vi "MDO32_2-2-Channel_V2.vi"() -> ()   [LabVIEW 2015]
uses:
  <vilib>/Utility/file.llb/Write Delimited Spreadsheet (string).vi
  <vilib>/Utility/file.llb/Write Delimited Spreadsheet (DBL).vi
panel:
  out "Iteration Running":bool
  out "Sample 4 Saved":bool
  out "Sample 3 Saved":bool
  out "Sample 2 Saved":bool
  out "Sample 1 Saved":bool
  in  "Test Name":string="TEST_NAME"
  in  "File Path Control":path
  in  "Temperature cDAQ1Mod1":tag="cDAQ1Mod1"
  in  "Oscilliscope MDO32_2":refnum<visa-resource-name>="MDO32_2"
  out "Iteration Number":i32
  out "Start Time and Date":timestamp
  in  "Stop":bool
  in  "Wait Time (s)":dbl=10.0
  in  "Oscilliscope MDO32_1":refnum<visa-resource-name>="MDO32_1"
  # "Test Settings"
  # "Test Info and Status"
  # "ENSURE THAT USBs ARE PLUGGED IN. DATA WILL NOT SAVE WITHOUT IT.\n\nUSB 1 GOES INTO OSC 1\nUSB 2 GOES INTO OSC 2\n\nPROGRAM WILL GET STUCK IF DEVICES ARE NOT CONNECTED OR SET UP APPROPRIATELY"
  # "CLICK STOP BUTTON ONLY ONCE\nIt takes time to stop as the loop needs to complete the current iteration and one more full iteration before it stops."
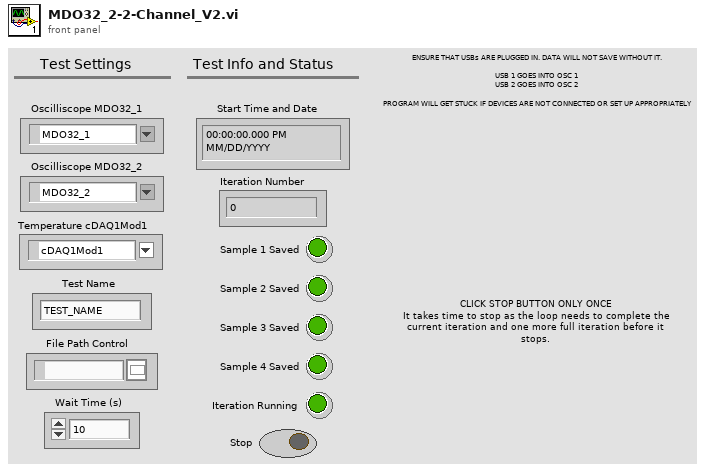
[diagram p1: front panel]
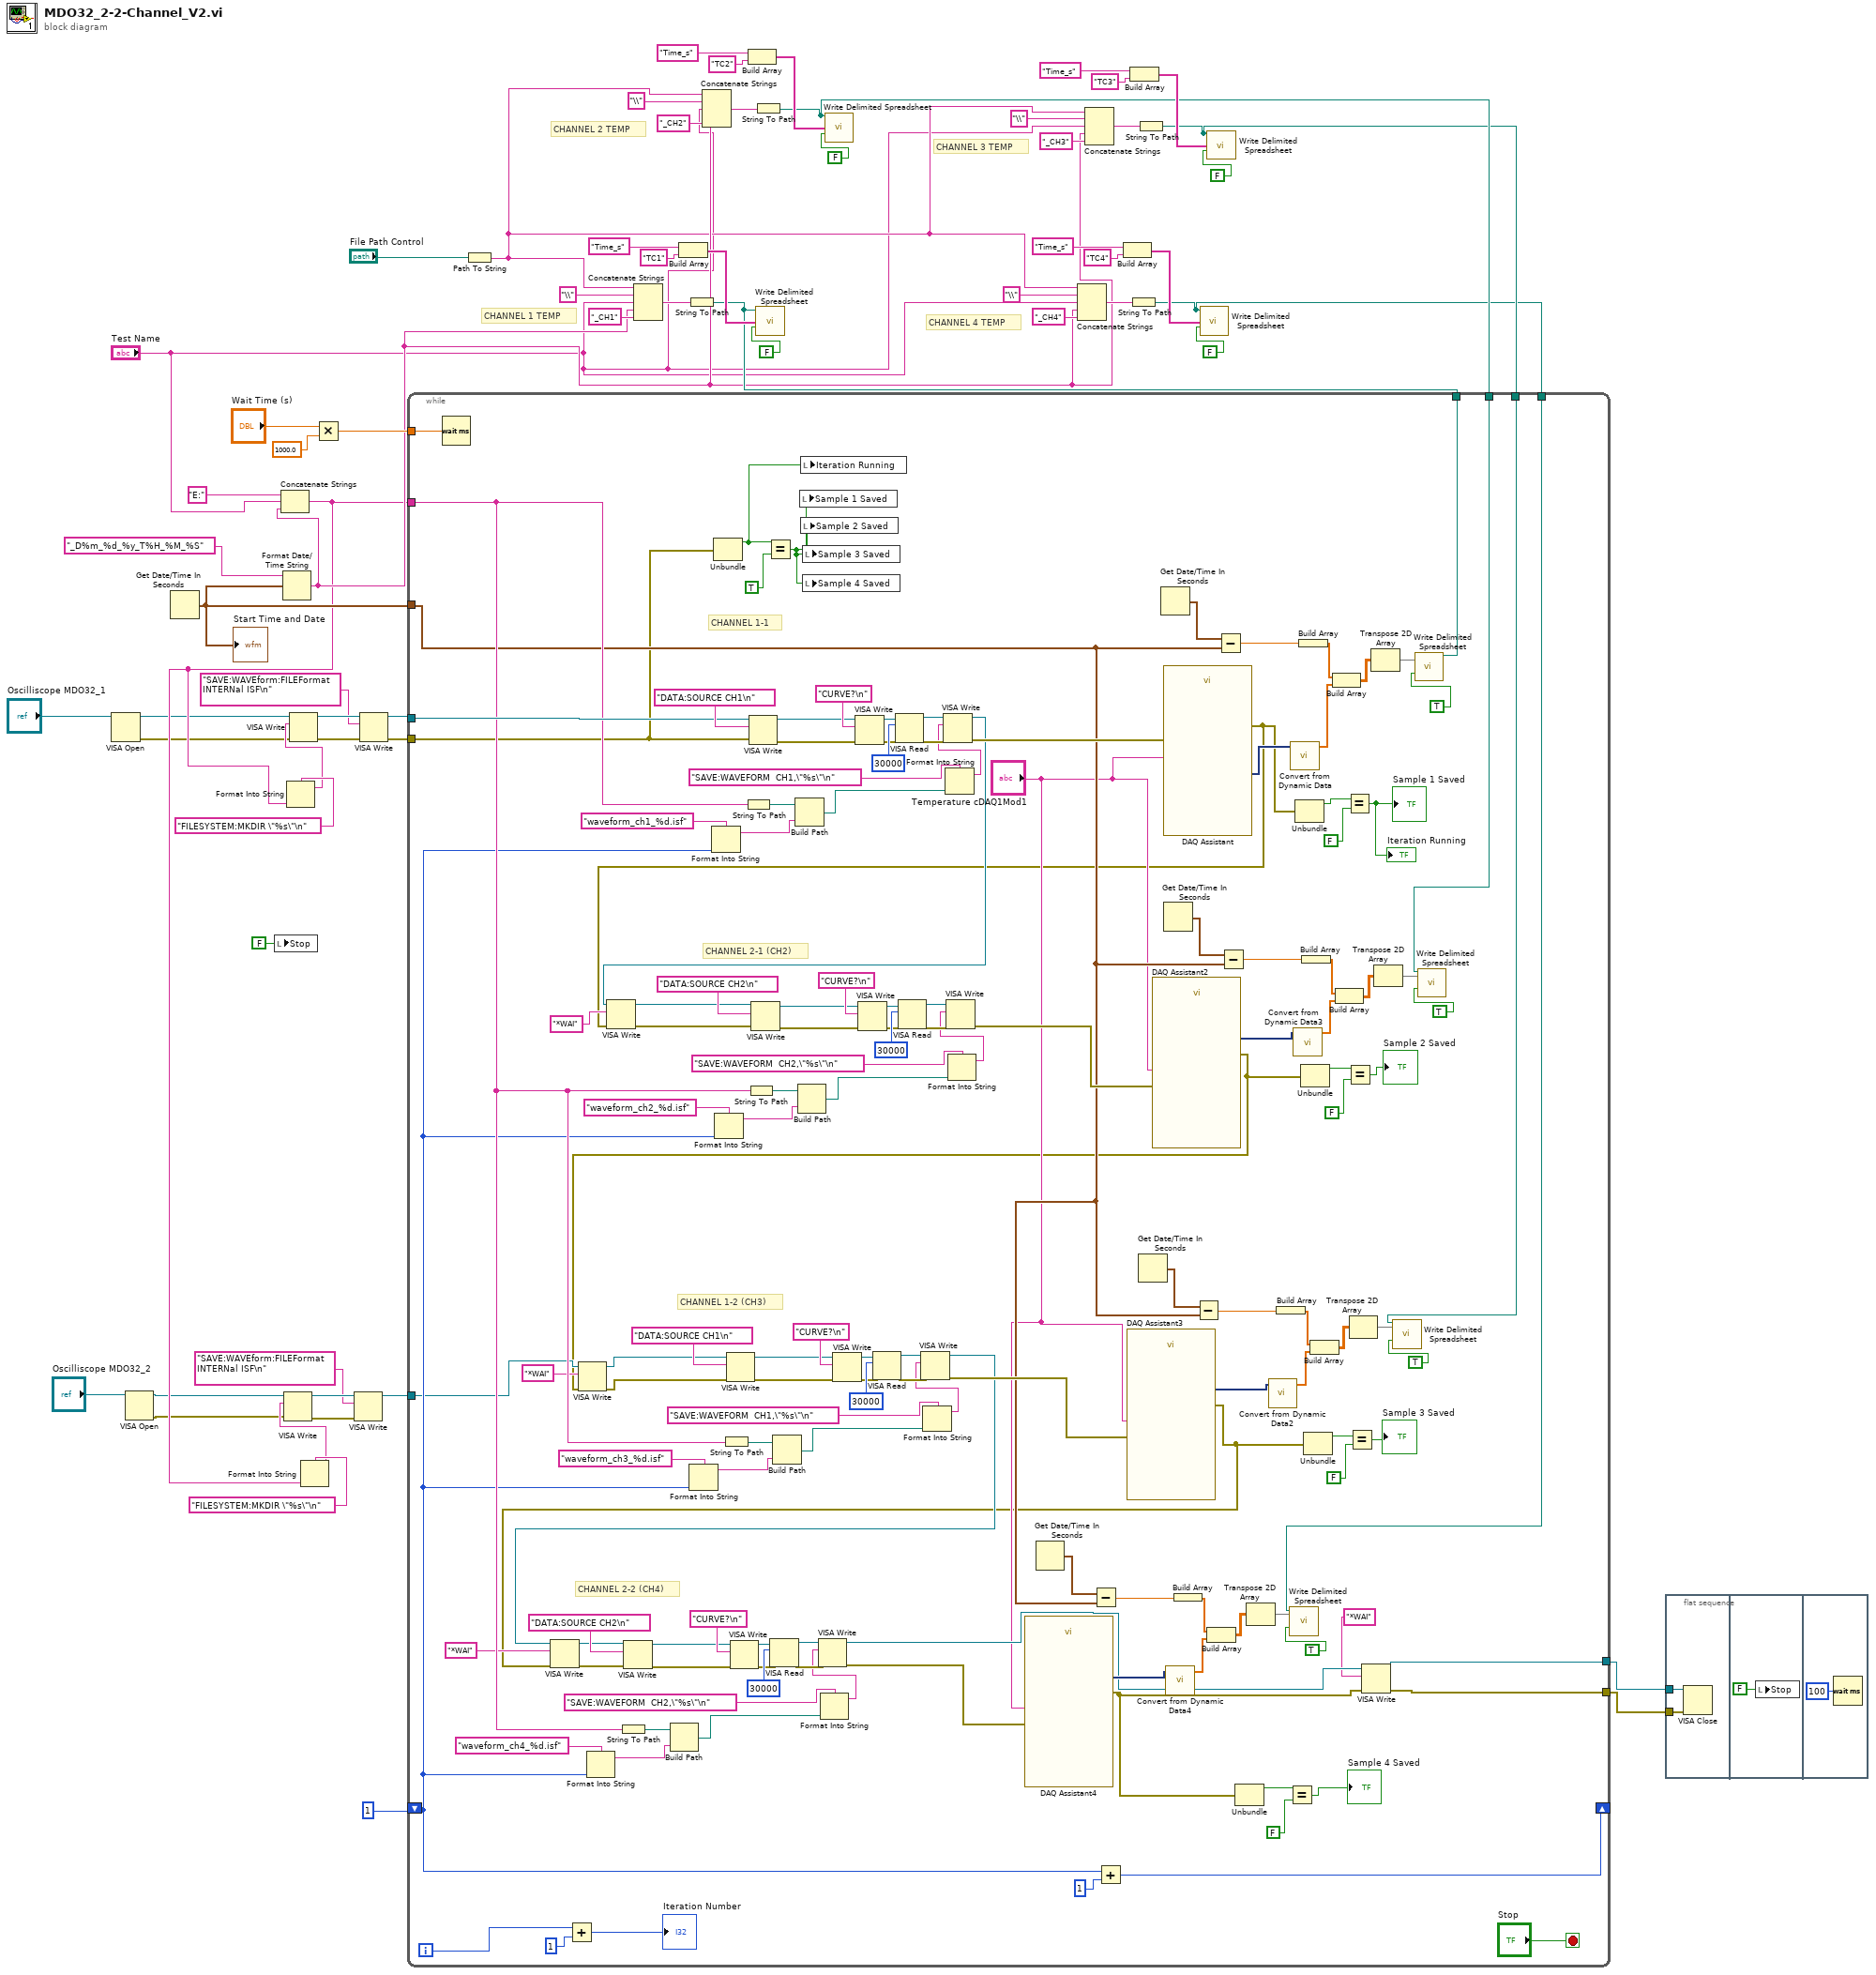
[diagram p0: block diagram]
diagram:
  # "CHANNEL 3 TEMP"
  # "CHANNEL 2 TEMP"
  # "CHANNEL 4 TEMP"
  # "CHANNEL 1 TEMP"
  n1 = VISA Open(VISA resource name="Oscilliscope MDO32_1") -> (VISA resource name=w8:refnum<visa-resource-name>, error out=w9:errorcluster)  [unwired: 4 in]
  n2 = VISA Open(VISA resource name="Oscilliscope MDO32_2") -> (VISA resource name=w6:refnum<visa-resource-name>, error out=w5:errorcluster)  [unwired: 4 in]
  n3 = Get Date/Time In Seconds() -> (seconds since 1Jan1904=w50:timestamp)
  "Start Time and Date" <- w50
  n4 = local write "Stop"(FALSE ("Stop")) -> ()
  n5 = Format Date/Time String(time format string (%c)="_D%m_%d_%y_T%H_%M_%S", seconds (now)=w50) -> (date/time string=w22:string)  [unwired: 1 in]
  n6 = Concatenate Strings("E:", "Test Name", w22) -> (w16:string)
  n7 = Format Into String(format string="FILESYSTEM:MKDIR \"%s\"\n", w16) -> (resulting string=w59:string)  [unwired: 2 in, 1 out]
  n8 = VISA Write(VISA resource name=w8, write buffer=w59, error in (no error)=w9) -> (VISA resource name out=w48:refnum<visa-resource-name>, error out=w49:errorcluster)  [unwired: 1 out]
  n9 = Format Into String(format string="FILESYSTEM:MKDIR \"%s\"\n", w16) -> (resulting string=w20:string)  [unwired: 2 in, 1 out]
  n10 = VISA Write(VISA resource name=w6, write buffer=w20, error in (no error)=w5) -> (VISA resource name out=w18:refnum<visa-resource-name>, error out=w19:errorcluster)  [unwired: 1 out]
  n11 = Multiply(x="Wait Time (s)", y=1000.0) -> (x*y=w62:dbl)
  n12 = VISA Write(VISA resource name=w18, write buffer="SAVE:WAVEform:FILEFormat INTERNal ISF\n", error in (no error)=w19) -> (VISA resource name out=w15:refnum<visa-resource-name>)  [unwired: 2 out]
  n13 = VISA Write(VISA resource name=w48, write buffer="SAVE:WAVEform:FILEFormat INTERNal ISF\n", error in (no error)=w49) -> (VISA resource name out=w47:refnum<visa-resource-name>, error out=w46:errorcluster)  [unwired: 1 out]
  n14 = Path To String(path="File Path Control") -> (string=w2:string)
  n15 = Concatenate Strings(w2, "\\" ("string"), "Test Name", w22, "_CH1" ("string")) -> (w58:string)
  n16 = Build Array("Time_s", "TC1") -> (w54:string[])
  n17 = String To Path(string=w58) -> (path=w53:path)
  n18 = Concatenate Strings(w2, "\\" ("string"), "Test Name", w22, "_CH2" ("string")) -> (w36:string)
  n19 = Build Array("Time_s", "TC2") -> (w32:string[])
  n20 = String To Path(string=w36) -> (path=w14:path)
  n21 = call-poly <vilib>:"Write Delimited Spreadsheet.vi"("file path (dialog if empty)"=w53, "1D data"=w54, "append to file? (F)"=FALSE ("append to file? (new file:F)")) -> ()  [unwired: 11 in, 2 out]
  n22 = call-poly <vilib>:"Write Delimited Spreadsheet.vi"("file path (dialog if empty)"=w14, "1D data"=w32, "append to file? (F)"=FALSE ("append to file? (new file:F)")) -> ()  [unwired: 11 in, 2 out]
  n23 = Concatenate Strings(w2, "\\" ("string"), "Test Name", w22, "_CH4" ("string")) -> (w44:string)
  n24 = Concatenate Strings(w2, "\\" ("string"), "Test Name", w22, "_CH3" ("string")) -> (w29:string)
  n25 = Build Array("Time_s", "TC4") -> (w40:string[])
  n26 = String To Path(string=w44) -> (path=w12:path)
  n27 = Build Array("Time_s", "TC3") -> (w25:string[])
  n28 = String To Path(string=w29) -> (path=w13:path)
  n29 = while {
    shift-right: [w207] -> _
    shift-left: 1 -> [w104]
    tunnel: w47 -> [w205]
    tunnel: w46 -> [w70]
    tunnel: w16 -> [w107]
    tunnel: w62 -> [w202]
    tunnel: w53 -> [w191]
    tunnel: w50 -> [w105]
    tunnel: w15 -> [w98]
    tunnel: w14 -> [w133]
    tunnel: w13 -> [w132]
    tunnel: w12 -> [w106]
    tunnel: [w90] -> w11
    tunnel: [w72] -> w10
    i -> [w160]
    stop <- "Stop" stop-if-true
    # "CHANNEL 2-2 (CH4)"
    # "CHANNEL 1-2 (CH3)"
    # "CHANNEL 2-1 (CH2)"
    # "CHANNEL 1-1"
    n30 = Wait (ms)(milliseconds to wait=w202) -> ()  [unwired: 1 out]
    n31 = Add(x=w160, y=1) -> (x+y=→"Iteration Number":i32)
    n32 = Format Into String(format string="waveform_ch4_%d.isf", w104) -> (resulting string=w123:string)  [unwired: 2 in, 1 out]
    n33 = String To Path(string=w107) -> (path=w122:path)
    n34 = Build Path(base path=w122, name or relative path=w123) -> (appended path=w121:path)
    n35 = Format Into String(format string="waveform_ch3_%d.isf", w104) -> (resulting string=w149:string)  [unwired: 2 in, 1 out]
    n36 = Format Into String(format string="waveform_ch1_%d.isf", w104) -> (resulting string=w204:string)  [unwired: 2 in, 1 out]
    n37 = Unbundle(w70) -> ("status"=w68:bool)  [unwired: 2 out]
    n38 = Format Into String(format string="waveform_ch2_%d.isf", w104) -> (resulting string=w179:string)  [unwired: 2 in, 1 out]
    n39 = String To Path(string=w107) -> (path=w148:path)
    n40 = String To Path(string=w107) -> (path=w203:path)
    n41 = String To Path(string=w107) -> (path=w178:path)
    n42 = VISA Write(VISA resource name=w205, write buffer="DATA:SOURCE CH1\n", error in (no error)=w70) -> (VISA resource name out=w189:refnum<visa-resource-name>, error out=w188:errorcluster)  [unwired: 1 out]
    n43 = Equal?(x=w68, y=TRUE) -> (x = y?=w71:bool)
    n44 = Build Path(base path=w148, name or relative path=w149) -> (appended path=w147:path)
    n45 = Build Path(base path=w203, name or relative path=w204) -> (appended path=w201:path)
    n46 = Build Path(base path=w178, name or relative path=w179) -> (appended path=w177:path)
    n47 = local write "Sample 1 Saved"(w71) -> ()
    n48 = local write "Iteration Running"(w68) -> ()
    n49 = local write "Sample 2 Saved"(w71) -> ()
    n50 = local write "Sample 3 Saved"(w71) -> ()
    n51 = local write "Sample 4 Saved"(w71) -> ()
    n52 = Format Into String(format string="SAVE:WAVEFORM  CH2,\"%s\"\n", w121) -> (resulting string=w119:string)  [unwired: 2 in, 1 out]
    n53 = VISA Write(VISA resource name=w189, write buffer="CURVE?\n", error in (no error)=w188) -> (VISA resource name out=w212:refnum<visa-resource-name>, error out=w211:errorcluster)  [unwired: 1 out]
    n54 = VISA Read(VISA resource name=w212, byte count=u32 30000, error in (no error)=w211) -> (VISA resource name out=w209:refnum<visa-resource-name>, error out=w208:errorcluster)  [unwired: 2 out]
    n55 = Format Into String(format string="SAVE:WAVEFORM  CH1,\"%s\"\n", w147) -> (resulting string=w145:string)  [unwired: 2 in, 1 out]
    n56 = Format Into String(format string="SAVE:WAVEFORM  CH1,\"%s\"\n", w201) -> (resulting string=w199:string)  [unwired: 2 in, 1 out]
    n57 = VISA Write(VISA resource name=w209, write buffer=w199, error in (no error)=w208) -> (VISA resource name out=w103:refnum<visa-resource-name>, error out=w165:errorcluster)  [unwired: 1 out]
    n58 = Format Into String(format string="SAVE:WAVEFORM  CH2,\"%s\"\n", w177) -> (resulting string=w175:string)  [unwired: 2 in, 1 out]
    n59 = Get Date/Time In Seconds() -> (seconds since 1Jan1904=w118:timestamp)
    n60 = Subtract(x=w118, y=w105) -> (x-y=w112:dbl)
    n61 = Add(x=w104, y=1) -> (x+y=w207:i32)
    n62 = Get Date/Time In Seconds() -> (seconds since 1Jan1904=w144:timestamp)
    n63 = Get Date/Time In Seconds() -> (seconds since 1Jan1904=w197:timestamp)
    n64 = call "DAQ Assistant"("error in"=w165, "device name"="Temperature cDAQ1Mod1") -> ("data"=w198:dynamicdata, "error out"=w87:errorcluster)  [unwired: 15 in, 1 out]
    n65 = VISA Write(VISA resource name=w103, write buffer="*WAI", error in (no error)=w87) -> (VISA resource name out=w101:refnum<visa-resource-name>, error out=w100:errorcluster)  [unwired: 1 out]
    n66 = VISA Write(VISA resource name=w101, write buffer="DATA:SOURCE CH2\n", error in (no error)=w100) -> (VISA resource name out=w167:refnum<visa-resource-name>, error out=w166:errorcluster)  [unwired: 1 out]
    n67 = VISA Write(VISA resource name=w167, write buffer="CURVE?\n", error in (no error)=w166) -> (VISA resource name out=w185:refnum<visa-resource-name>, error out=w184:errorcluster)  [unwired: 1 out]
    n68 = VISA Read(VISA resource name=w185, byte count=u32 30000, error in (no error)=w184) -> (VISA resource name out=w182:refnum<visa-resource-name>, error out=w181:errorcluster)  [unwired: 2 out]
    n69 = VISA Write(VISA resource name=w182, write buffer=w175, error in (no error)=w181) -> (error out=w164:errorcluster)  [unwired: 2 out]
    n70 = call "DAQ Assistant2"("error in"=w164, "device name"="Temperature cDAQ1Mod1") -> ("data"=w159:dynamicdata, "error out"=w86:errorcluster)  [unwired: 15 in, 1 out]
    n71 = VISA Write(VISA resource name=w98, write buffer="*WAI", error in (no error)=w86) -> (VISA resource name out=w97:refnum<visa-resource-name>, error out=w99:errorcluster)  [unwired: 1 out]
    n72 = VISA Write(VISA resource name=w97, write buffer="DATA:SOURCE CH1\n", error in (no error)=w99) -> (VISA resource name out=w137:refnum<visa-resource-name>, error out=w136:errorcluster)  [unwired: 1 out]
    n73 = VISA Write(VISA resource name=w137, write buffer="CURVE?\n", error in (no error)=w136) -> (VISA resource name out=w155:refnum<visa-resource-name>, error out=w154:errorcluster)  [unwired: 1 out]
    n74 = VISA Read(VISA resource name=w155, byte count=u32 30000, error in (no error)=w154) -> (VISA resource name out=w152:refnum<visa-resource-name>, error out=w151:errorcluster)  [unwired: 2 out]
    n75 = VISA Write(VISA resource name=w152, write buffer=w145, error in (no error)=w151) -> (VISA resource name out=w95:refnum<visa-resource-name>, error out=w135:errorcluster)  [unwired: 1 out]
    n76 = call "DAQ Assistant3"("error in"=w135, "device name"="Temperature cDAQ1Mod1") -> ("data"=w134:dynamicdata, "error out"=w85:errorcluster)  [unwired: 15 in, 1 out]
    n77 = VISA Write(VISA resource name=w95, write buffer="*WAI", error in (no error)=w85) -> (VISA resource name out=w93:refnum<visa-resource-name>, error out=w94:errorcluster)  [unwired: 1 out]
    n78 = VISA Write(VISA resource name=w93, write buffer="DATA:SOURCE CH2\n", error in (no error)=w94) -> (VISA resource name out=w111:refnum<visa-resource-name>, error out=w110:errorcluster)  [unwired: 1 out]
    n79 = VISA Write(VISA resource name=w111, write buffer="CURVE?\n", error in (no error)=w110) -> (VISA resource name out=w129:refnum<visa-resource-name>, error out=w128:errorcluster)  [unwired: 1 out]
    n80 = VISA Read(VISA resource name=w129, byte count=u32 30000, error in (no error)=w128) -> (VISA resource name out=w126:refnum<visa-resource-name>, error out=w125:errorcluster)  [unwired: 2 out]
    n81 = VISA Write(VISA resource name=w126, write buffer=w119, error in (no error)=w125) -> (VISA resource name out=w91:refnum<visa-resource-name>, error out=w109:errorcluster)  [unwired: 1 out]
    n82 = call "DAQ Assistant4"("error in"=w109, "device name"="Temperature cDAQ1Mod1") -> ("data"=w108:dynamicdata, "error out"=w84:errorcluster)  [unwired: 15 in, 1 out]
    n83 = Get Date/Time In Seconds() -> (seconds since 1Jan1904=w174:timestamp)
    n84 = call "Convert from Dynamic Data4"("Dynamic Data Type"=w108) -> ("Array"=w117:dbl[])  [unwired: 3 in]
    n85 = Build Array(w112) -> (w116:dbl[])
    n86 = Subtract(x=w144, y=w105) -> (x-y=w138:dbl)
    n87 = Build Array(w116, w117) -> (w115:dbl[][])
    n88 = Subtract(x=w197, y=w105) -> (x-y=w190:dbl)
    n89 = Subtract(x=w174, y=w105) -> (x-y=w168:dbl)
    n90 = Unbundle(w84) -> ("status"=w78:bool)  [unwired: 2 out]
    n91 = Transpose 2D Array(2D array=w115) -> (transposed array=w114:dbl[][])
    n92 = call "Convert from Dynamic Data2"("Dynamic Data Type"=w134) -> ("Array"=w143:dbl[])  [unwired: 3 in]
    n93 = Build Array(w138) -> (w142:dbl[])
    n94 = Equal?(x=w78, y=FALSE) -> (x = y?=→"Sample 4 Saved":bool)
    n95 = call-poly <vilib>:"Write Delimited Spreadsheet.vi"("file path (dialog if empty)"=w106, "2D data"=w114, "append to file? (F)"=TRUE) -> ()  [unwired: 11 in, 2 out]
    n96 = call "Convert from Dynamic Data"("Dynamic Data Type"=w198) -> ("Array"=w196:dbl[])  [unwired: 3 in]
    n97 = call "Convert from Dynamic Data3"("Dynamic Data Type"=w159) -> ("Array"=w173:dbl[])  [unwired: 3 in]
    n98 = Unbundle(w87) -> ("status"=w83:bool)  [unwired: 2 out]
    n99 = Build Array(w190) -> (w195:dbl[])
    n100 = Unbundle(w86) -> ("status"=w75:bool)  [unwired: 2 out]
    n101 = Build Array(w168) -> (w172:dbl[])
    n102 = Unbundle(w85) -> ("status"=w77:bool)  [unwired: 2 out]
    n103 = Build Array(w142, w143) -> (w141:dbl[][])
    n104 = Build Array(w195, w196) -> (w194:dbl[][])
    n105 = Build Array(w172, w173) -> (w171:dbl[][])
    n106 = Equal?(x=w83, y=FALSE) -> (x = y?=→"Sample 1 Saved" →"Iteration Running":bool)
    n107 = Equal?(x=w75, y=FALSE) -> (x = y?=→"Sample 2 Saved":bool)
    n108 = Equal?(x=w77, y=FALSE) -> (x = y?=→"Sample 3 Saved":bool)
    n109 = Transpose 2D Array(2D array=w141) -> (transposed array=w140:dbl[][])
    n110 = VISA Write(VISA resource name=w91, write buffer="*WAI", error in (no error)=w84) -> (VISA resource name out=w90:refnum<visa-resource-name>, error out=w72:errorcluster)  [unwired: 1 out]
    n111 = Transpose 2D Array(2D array=w194) -> (transposed array=w193:dbl[][])
    n112 = Transpose 2D Array(2D array=w171) -> (transposed array=w170:dbl[][])
    n113 = call-poly <vilib>:"Write Delimited Spreadsheet.vi"("file path (dialog if empty)"=w132, "2D data"=w140, "append to file? (F)"=TRUE) -> ()  [unwired: 11 in, 2 out]
    n114 = call-poly <vilib>:"Write Delimited Spreadsheet.vi"("file path (dialog if empty)"=w191, "2D data"=w193, "append to file? (F)"=TRUE) -> ()  [unwired: 11 in, 2 out]
    n115 = call-poly <vilib>:"Write Delimited Spreadsheet.vi"("file path (dialog if empty)"=w133, "2D data"=w170, "append to file? (F)"=TRUE) -> ()  [unwired: 11 in, 2 out]
  }
  n116 = call-poly <vilib>:"Write Delimited Spreadsheet.vi"("file path (dialog if empty)"=w12, "1D data"=w40, "append to file? (F)"=FALSE ("append to file? (new file:F)")) -> ()  [unwired: 11 in, 2 out]
  n117 = call-poly <vilib>:"Write Delimited Spreadsheet.vi"("file path (dialog if empty)"=w13, "1D data"=w25, "append to file? (F)"=FALSE ("append to file? (new file:F)")) -> ()  [unwired: 11 in, 2 out]
  n118 = flat-sequence {
    tunnel: w11 -> [w216]
    tunnel: w10 -> [w215]
    frame #0 {
      n119 = VISA Close(VISA resource name=w216, error in (no error)=w215) -> ()  [unwired: 1 out]
    }
    frame #1 {
      n120 = local write "Stop"(FALSE ("Stop")) -> ()
    }
    frame #2 {
      n121 = Wait (ms)(milliseconds to wait=u32 100) -> ()  [unwired: 1 out]
    }
  }
